vi "InitAll.vi"(3 "任务":i32[](array[numeric])) -> (0 "error IO":errorcluster caption="error out")   [LabVIEW 2012]
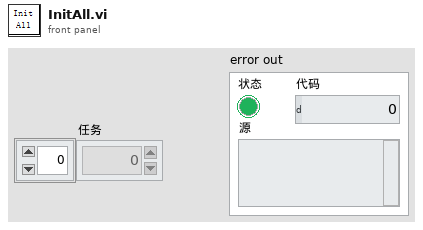
[diagram p1: front panel]
types:
  T1 = enum16{"功率测量", "能量测量", "光谱测量", "时间波形", "近远场", "偏振"}
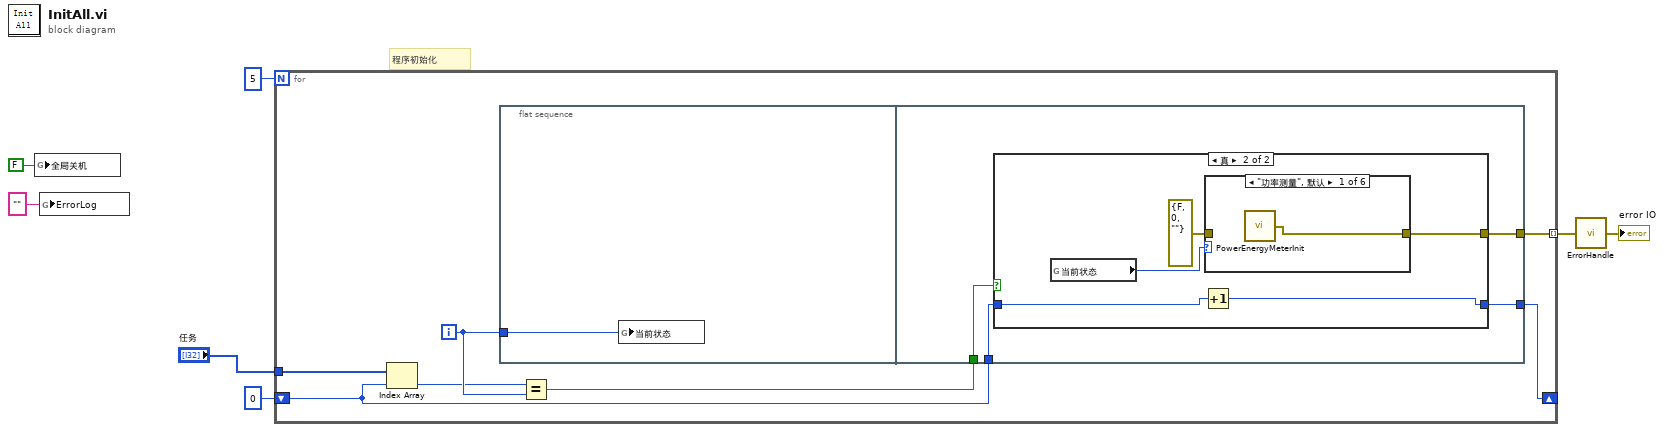
[diagram p0: block diagram]
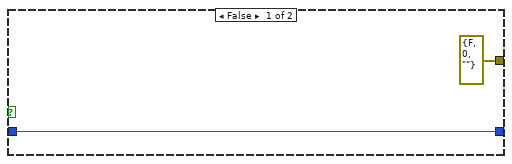
[diagram p2: hidden frame]
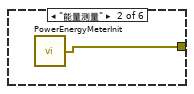
[diagram p3: hidden frame]
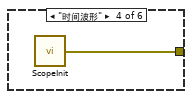
[diagram p5: hidden frame]
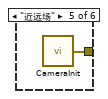
[diagram p6: hidden frame]
diagram:
  # "程序初始化"
  n1 = global write "参数.vi" "全局关机"(FALSE ("全局关机")) -> ()
  n2 = global write "参数.vi" "ErrorLog"("" ("ErrorLog")) -> ()
  n3 = for {
    N: 5 -> [_]
    tunnel: "任务" -> [w14]
    shift-right: [w10] -> _
    shift-left: 0 -> [w8]
    tunnel: [w9] -> w5 mode=indexing
    i -> [w13]
    n4 = Index Array(array=w14, index=w8) -> (element=w11:i32)
    n5 = flat-sequence {
      tunnel: w13 -> [w15]
      tunnel: w12 -> [w19]
      tunnel: w8 -> [w16]
      tunnel: [w18] -> w10
      tunnel: [w17] -> w9
      frame #0 {
        n6 = global write "参数.vi" "当前状态"(w15) -> ()
      }
      frame #1 {
        n7 = case shown="真" w19 {
          tunnel: w16 -> [w20 w26]
          tunnel: [w20 w25] -> w18
          tunnel: [errorcluster {"status"=FALSE, "code"=0, "source"=""} ("error out") w22] -> w17
          frame False {
          }
          frame True {
            n8 = global read "参数.vi" "当前状态"() -> (w24:T1)
            n9 = Increment(x=w26) -> (x+1=w25:i32)
            n10 = case shown="\"功率测量\", 默认" w24 {
              tunnel: [w27 w28 w29 w30 w31 w32] -> w22
              tunnel: errorcluster {"status"=FALSE, "code"=0, "source"=""} ("error out") -> [_ _ w29 _ _ w32]
              frame "功率测量", Default {
                n11 = call "PowerEnergyMeterInit.vi"() -> ("错误输出"=w27:errorcluster)  [unwired: 1 in]
              }
              frame "能量测量" {
                n12 = call "PowerEnergyMeterInit.vi"() -> ("错误输出"=w28:errorcluster)  [unwired: 1 in]
              }
              frame "光谱测量" {
              }
              frame "时间波形" {
                n13 = call "ScopeInit.vi"() -> ("error out"=w30:errorcluster)  [unwired: 1 in]
              }
              frame "近远场" {
                n14 = call "CameraInit.vi"() -> ("error out"=w31:errorcluster)  [unwired: 1 in]
              }
              frame "偏振" {
              }
            }
          }
        }
      }
    }
    n15 = Equal?(x=w11, y=w13) -> (x = y?=w12:bool)
  }
  n16 = call "ErrorHandle.vi"("Error"=w5) -> ("error IO"=→"error IO":errorcluster)
